vi "Agilent_Initialize.vi"(8 "error in (no error)":errorcluster, 9 "Reset? (T: Yes)":bool=TRUE, 10 "ID Query? (T: Yes)":bool=TRUE, 11 "VISA resource name":refnum<visa-resource-name>) -> (0 "error out":errorcluster, 3 "VISA resource name out":refnum<visa-resource-name>)   [LabVIEW 2020]
doc: "Establishes communication with the instrument and optionally performs an instrument identification query and/or an instrument reset. It also places the instrument in a default state needed for other instrument driver operations. Therefore, call this VI before calling other instrument driver VIs for this instrument. Generally, you need to call the <B>Initialize VI</B> only once at the beginning of an application."
panel:
  # "(c) 2009 National Instruments.  ALL RIGHTS RESERVED."
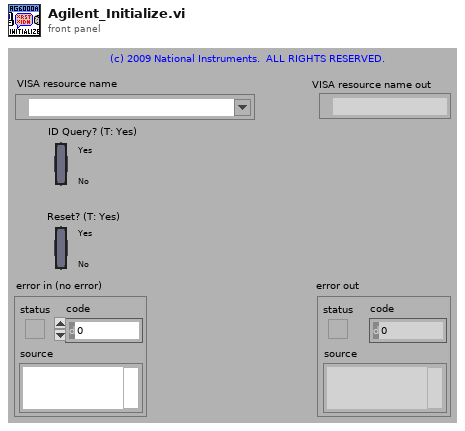
[diagram p1: front panel]
types:
  T1 = cluster{"Status":bool, "Code":i32, "Source (VI Name)":string}
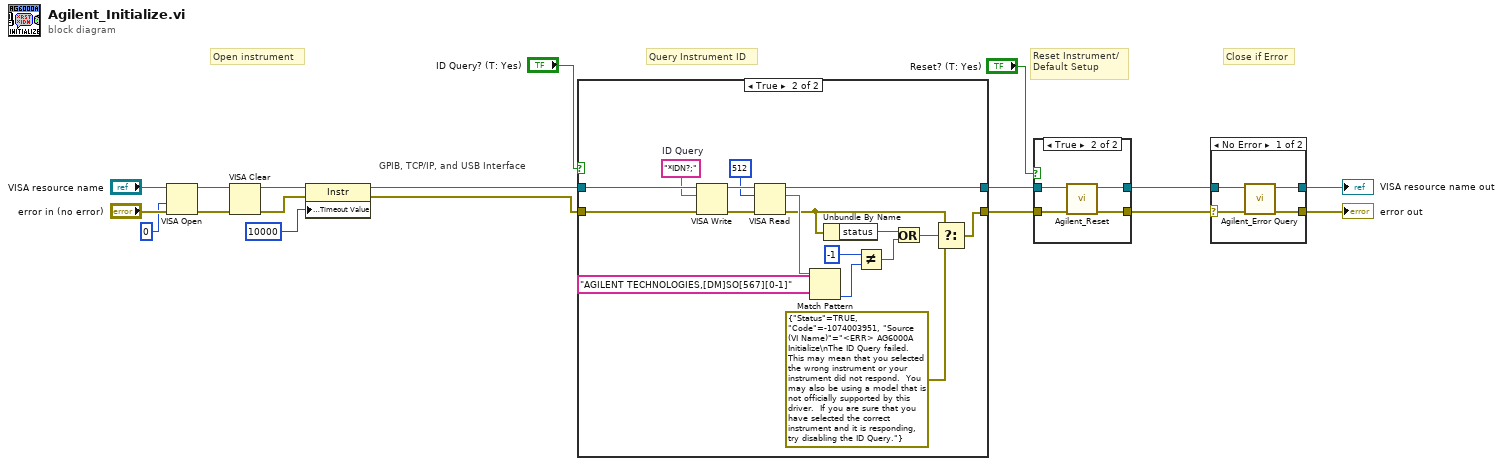
[diagram p0: block diagram]
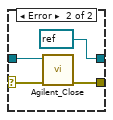
[diagram p2: hidden frame]
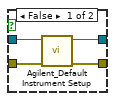
[diagram p3: hidden frame]
diagram:
  # "GPIB, TCP/IP, and USB Interface"
  # "Close if Error"
  # "Query Instrument ID"
  # "Reset Instrument/\nDefault Setup"
  # "Open instrument"
  n1 = VISA Open(access mode=u32 0, error in (no error)="error in (no error)", VISA resource name="VISA resource name") -> (VISA resource name=w8:refnum<visa-resource-name>, error out=w7:errorcluster)  [unwired: 2 in]
  n2 = VISA Clear(VISA resource name=w8, error in (no error)=w7) -> (VISA resource name out=w6:refnum<visa-resource-name>, error out=w5:errorcluster)
  n3 = property on="Property Node" class="Instr"(reference=w6, error in=w5, "General Settings:Timeout Value"=u32 10000) -> (reference out=w11:refnum<visa-resource-name>, error out=w10:errorcluster)
  n4 = case shown="True" "ID Query? (T: Yes)" {
    tunnel: [w19 w37] -> w17
    tunnel: [w20 w34] -> w18
    tunnel: w11 -> [w20 w35]
    tunnel: w10 -> [w19 w36]
    frame False {
    }
    frame True {
      w22 = "*IDN?;"  # ID Query
      n5 = VISA Write(VISA resource name=w35, write buffer=w22, error in (no error)=w36) -> (VISA resource name out=w31:refnum<visa-resource-name>, error out=w29:errorcluster)  [unwired: 1 out]
      n6 = VISA Read(VISA resource name=w31, byte count=u32 512, error in (no error)=w29) -> (VISA resource name out=w34:refnum<visa-resource-name>, read buffer=w32:string, error out=w30:errorcluster)  [unwired: 1 out]
      n7 = Match Pattern(string=w32, regular expression="AGILENT TECHNOLOGIES,[DM]SO[567][0-1]") -> (offset past match=w24:i32)  [unwired: 1 in, 3 out]
      n8 = Unbundle By Name(w30) -> ("status"=w27:bool)
      n9 = Not Equal?(x=-1, y=w24) -> (x != y?=w33:bool)
      n10 = Or(x=w27, y=w33) -> (x .or. y?=w28:bool)
      n11 = Select(t=w30, s=w28, f=T1 {"Status"=TRUE, "Code"=-1074003951, "Source (VI Name)"="<ERR> AG6000A Initialize\nThe ID Query failed.  This may mean that you selected the wrong instrument or your instrument did not respond.  You may also be using a model that is not officially supported by this driver.  If you are sure that you have selected the correct instrument and it is responding, try disabling the ID Query."}) -> (s? t:f=w37:T1)
    }
  }
  n12 = case shown="True" "Reset? (T: Yes)" {
    tunnel: w17 -> [w40 w42]
    tunnel: [w39 w45] -> w1
    tunnel: w18 -> [w41 w43]
    tunnel: [w38 w44] -> w2
    frame False {
      n13 = call "Agilent_Default Instrument Setup.vi"("error in (no error)"=w40, "VISA resource name"=w41) -> ("error out"=w39:errorcluster, "VISA resource name out"=w38:refnum<visa-resource-name>)  [unwired: 8 in]
    }
    frame True {
      n14 = call "Agilent_Reset.vi"("error in (no error)"=w42, "VISA resource name"=w43) -> ("error out"=w45:errorcluster, "VISA resource name out"=w44:refnum<visa-resource-name>)  [unwired: 8 in]
    }
  }
  n15 = case shown="No Error" w1 {
    selector: w1 -> [w47 w51]
    tunnel: w2 -> [w46 w52]
    tunnel: [w49 refnum<visa-resource-name> refnum ("VISA resource name out")] -> w4
    tunnel: [w48 w53] -> w3
    frame No Error {
      n16 = call "Agilent_Error Query.vi"("error in (no error)"=w47, "VISA resource name"=w46) -> ("error out"=w48:errorcluster, "VISA resource name out"=w49:refnum<visa-resource-name>)  [unwired: 6 in, 2 out]
    }
    frame Error {
      n17 = call "Agilent_Close.vi"("error in (no error)"=w51, "VISA resource name"=w52) -> ("error out"=w53:errorcluster)  [unwired: 9 in]
    }
  }
  "VISA resource name out" <- w4
  "error out" <- w3
